vi "pulse from memory 8spc_v2_test version.vi"(9 "referenses":T3={"clock x2"="IO Socket\\Data Clock 2x", "Memory In"="pulse on memory"}, 10 "start this pulse":bool, 11 "PDW":T1={"PW"=0, "frequency shift"=0.0, "amp"=0.9999923706054688, "mode type"=enum."CW", "mode depth"=0, "mode filter"=0, "phase shift"=0.0, "pulse shape filter"=0} {"frequency shift" format="%#_12f"}) -> (1 "free DDS":bool, 3 "IQ_out":T4[](array[typedef]))   [LabVIEW 2021]
uses:
  <instrlib>/_niInstr/DSP/v1/Shared/Public/IQ Data.ctl
  pdw.ctl
  CTL/mode_type.ctl
  <instrlib>/_niInstr/DSP/v1/FPGA/Public/Sub VIs/Data Conversion/U32 to IQ - 1 spc - S18.1.vi
  <instrlib>/FlexRIO/API/UsrFpgaDsp/v1/FPGA/HbInt/UsrFpgaDspHbIntIQ_8Cps_1xOC_BWper2_96dB.vi
  <instrlib>/FlexRIO/API/UsrFpgaDsp/v1/FPGA/HbInt/UsrFpgaDspHbIntIQ_4Cps_1xOC_BWper2_89dB.vi
  <instrlib>/FlexRIO/API/UsrFpgaDsp/v1/FPGA/HbInt/UsrFpgaDspHbIntIQ_2Cps_1xOC_BWper2_89dB.vi
  <instrlib>/FlexRIO/API/UsrFpgaDsp/v1/FPGA/HbInt/UsrFpgaDspHbIntIQ_1Spc_2xOC_BWper2_89dB.vi
  <instrlib>/FlexRIO/API/UsrFpgaDsp/v1/FPGA/HbInt/UsrFpgaDspHbIntIQ_2Spc_2xOC_BWper2_89dB.vi
  <instrlib>/FlexRIO/API/UsrFpgaDsp/v1/FPGA/HbInt/UsrFpgaDspHbIntIQ_4Spc_2xOC_BWper2_89dB.vi
  <instrlib>/_niInstr/DSP/v1/FPGA/Public/Sub VIs/Frequency Shift/Frequency Shift - 8 spc.vi
  <instrlib>/_niInstr/Basic Elements/v1/FPGA/Private/Count Up U16.vi
  <instrlib>/_niInstr/DSP/v1/Shared/niInstr DSP v1 Shared.lvlib
  <instrlib>/_niInstr/DSP/v1/FPGA/niInstr DSP v1 FPGA.lvlib
  <instrlib>/_niInstr/Basic Elements/v1/FPGA/niInstr Basic Elements v1 FPGA.lvlib
  <instrlib>/FlexRIO/API/UsrFpgaDsp/v1/FPGA/HbInt/UsrFpgaDsp HbInt v1 FPGA.lvlib
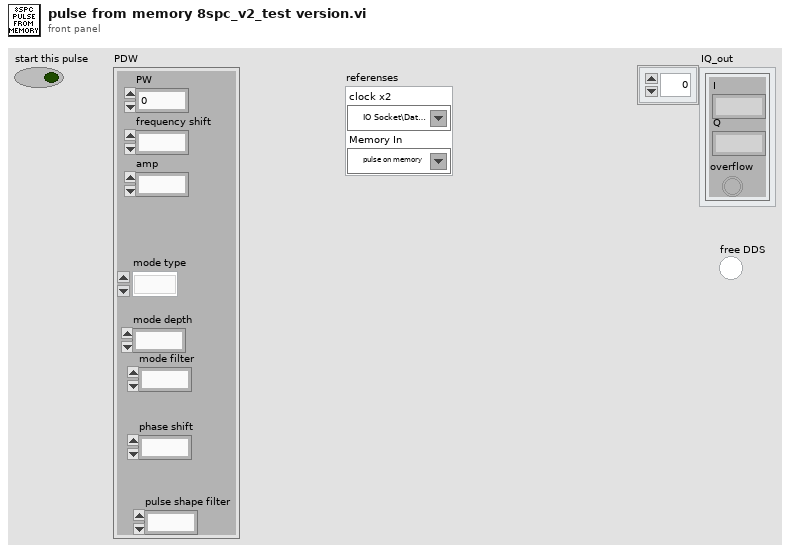
[diagram p1: front panel]
types:
  T1 = typedef "pdw.ctl" = cluster{"PW":u32, "frequency shift":fxp<+/-,48,0>, "amp":fxp<+/-,18,1>, "mode type":T2, "mode depth":u32, "mode filter":u8, "phase shift":fxp<+/-,16,1>, "pulse shape filter":u8}
  T2 = typedef "mode_type.ctl" = enum8{"CW", "from memory 1", "NC - cw", "LFM", "BPSK", "QPSK"}
  T3 = cluster{"clock x2":refnum<k21>, "Memory In":refnum<k21>}
  T4 = typedef "niInstr DSP v1 Shared.lvlib/IQ Data.ctl" = cluster{"I":fxp<+/-,18,1>, "Q":fxp<+/-,18,1>, "overflow":bool}
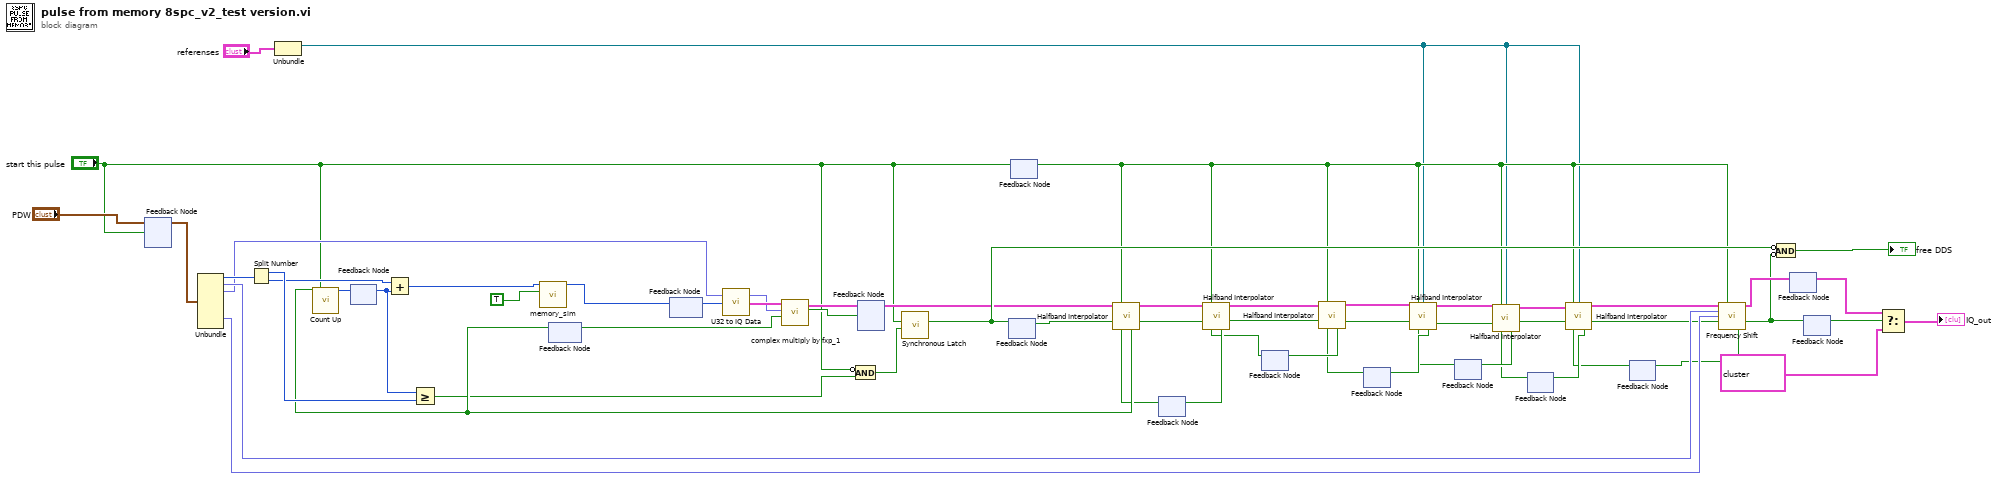
[diagram p0: block diagram]
diagram:
  n1 = feedback #1() -> (w51:T1)  [unwired: 1 in]
  n2 = feedback-in #1("PDW", "start this pulse") -> ()
  n3 = Unbundle(w51) -> ("PW"=w50:u32, "frequency shift"=w56:fxp<+/-,48,0>, "amp"=w44:fxp<+/-,18,1>, "phase shift"=w55:fxp<+/-,16,1>)  [unwired: 4 out]
  n4 = Split Number(x=w50) -> (hi(x)=w49:u16, lo(x)=w43:u16)
  n5 = Unbundle("referenses") -> ("clock x2"=w18:refnum<k21>)  [unwired: 1 out]
  n6 = feedback #2() -> (w41:u16)  [unwired: 1 in]
  n7 = Add(x=w43, y=w41) -> (x+y=w3:u16)
  n8 = Greater Or Equal?(x=w41, y=w49) -> (x >= y?=w16:bool)
  n9 = call "memory_sim.vi"("t-read;fwrite"=TRUE, "index"=w3) -> ("element out"=w2:u32)  [unwired: 8 in, 1 out]
  n10 = feedback #3() -> (w45:bool)  [unwired: 1 in]
  n11 = feedback #4() -> (w59:u32)  [unwired: 1 in]
  n12 = feedback-in #4(w2) -> ()
  n13 = call-poly <instrlib>:"U32 to IQ Data.vi"("U32 data"=w59) -> ("IQ data"=w47:T4)  [unwired: 14 in]
  n14 = call "complex multiply by fxp_1.vi"("input valid"=w45, "amp"=w44, "IQ data"=w47) -> ("data valid"=w48:bool, "output cluster"=w46:T4)  [unwired: 7 in]
  n15 = Compound Arithmetic op=AND(invert "start this pulse", w16) -> (w58:bool)
  n16 = feedback #5() -> (w24:T4)  [unwired: 1 in]
  n17 = feedback-in #5(w46, w48) -> ()
  n18 = call <instrlib>:"Synchronous Latch.vi"("clear"=w58, "set"="start this pulse") -> ("out"=w35:bool)  [unwired: 9 in]
  n19 = feedback #6() -> (w23:bool)  [unwired: 1 in]
  n20 = feedback-in #6(w35) -> ()
  n21 = feedback-in #7("start this pulse") -> ()
  n22 = feedback #7() -> (w19:bool)  [unwired: 1 in]
  n23 = feedback #8() -> (w4:bool)  [unwired: 1 in]
  n24 = call-poly "Halfband Interpolator.vi"("data in"=w24, "reset"=w19, "input valid"=w23, "ready for output (T)"=w4) -> ("data out"=w34:T4, "output valid"=w25:bool, "ready for input"=w20:bool)  [unwired: 9 in]
  n25 = call-poly <instrlib>:"Count Up.vi"("increment"=w20, "reset"="start this pulse") -> ("count out"=w42:u16)  [unwired: 13 in]
  n26 = feedback-in #2(w42) -> ()
  n27 = feedback-in #3(w20) -> ()
  n28 = feedback #9() -> (w13:bool)  [unwired: 1 in]
  n29 = call-poly "Halfband Interpolator.vi"("data in"=w34, "reset"=w19, "input valid"=w25, "ready for output (T)"=w13) -> ("data out"=w33:T4, "output valid"=w26:bool, "ready for input"=w15:bool)  [unwired: 9 in]
  n30 = feedback-in #8(w15) -> ()
  n31 = feedback #10() -> (w11:bool)  [unwired: 1 in]
  n32 = call-poly "Halfband Interpolator.vi"("data in"=w33, "reset"=w19, "input valid"=w26, "ready for output (T)"=w11) -> ("data out"=w32:T4, "output valid"=w27:bool, "ready for input"=w14:bool)  [unwired: 9 in]
  n33 = feedback-in #9(w14) -> ()
  n34 = feedback #11() -> (w9:bool)  [unwired: 1 in]
  n35 = call-poly "Halfband Interpolator.vi"("data in"=w32, "reset"=w19, "clk2x"=w18, "input valid"=w27, "ready for output (T)"=w9) -> ("data out"=w31:T4[], "output valid"=w28:bool, "ready for input"=w12:bool)  [unwired: 8 in]
  n36 = feedback-in #10(w12) -> ()
  n37 = feedback #12() -> (w7:bool)  [unwired: 1 in]
  n38 = call-poly "Halfband Interpolator.vi"("data in"=w31, "reset"=w19, "clk2x"=w18, "input valid"=w28, "ready for output (T)"=w7) -> ("data out"=w30:T4[], "output valid"=w29:bool, "ready for input"=w10:bool)  [unwired: 8 in]
  n39 = feedback-in #11(w10) -> ()
  n40 = feedback #13() -> (w5:bool)  [unwired: 1 in]
  n41 = call-poly "Halfband Interpolator.vi"("data in"=w30, "reset"=w19, "clk2x"=w18, "input valid"=w29, "ready for output (T)"=w5) -> ("data out"=w21:T4[], "output valid"=w22:bool, "ready for input"=w8:bool)  [unwired: 8 in]
  n42 = feedback-in #12(w8) -> ()
  n43 = call-poly <instrlib>:"Frequency Shift.vi"("data in"=w21, "reset"=w19, "frequency shift"=w56, "phase"=w55, "input valid"=w22) -> ("data out"=w40:T4[], "output valid"=w38:bool, "ready for input"=w6:bool)  [unwired: 7 in, 1 out]
  n44 = feedback-in #13(w6) -> ()
  n45 = Compound Arithmetic op=AND(invert w35, invert w38) -> (→"free DDS":bool)
  n46 = feedback #14() -> (w39:T4[])  [unwired: 1 in]
  n47 = feedback-in #14(w40) -> ()
  n48 = feedback #15() -> (w37:bool)  [unwired: 1 in]
  n49 = feedback-in #15(w38) -> ()
  n50 = Select(t=w39, s=w37, f=T4[] [{"I"=0.0, "Q"=0.0, "overflow"=FALSE}, {"I"=0.0, "Q"=0.0, "overflow"=FALSE}, {"I"=0.0, "Q"=0.0, "overflow"=FALSE}, {"I"=0.0, "Q"=0.0, "overflow"=FALSE}, {"I"=0.0, "Q"=0.0, "overflow"=FALSE}, {"I"=0.0, "Q"=0.0, "overflow"=FALSE}, {"I"=0.0, "Q"=0.0, "overflow"=FALSE}, {"I"=0.0, "Q"=0.0, "overflow"=FALSE}] ("data out")) -> (s? t:f=→"IQ_out":T4[])
